vi "add method.vi"   [LabVIEW 2013, in "vi modification tool.lvclass"]
uses:
  vi modification tool.lvclass
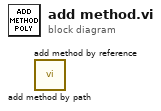
[diagram p0: block diagram]
diagram:
  n1 = call "add method by path.vi"() -> ()  [unwired: 10 in, 2 out]
  n2 = call "add method by reference.vi"() -> ()  [unwired: 10 in, 2 out]
